vi "MHM Get DLL Version.vi"(8 "error in (no error)":errorcluster) -> (0 "error out":errorcluster, 2 "pulDllVersion":u32[](array[numeric]), 3 "function return":u32)   [LabVIEW 2019, in "MHM_1SL_interface.lvlib"]
uses:
  MHM_1SL_interface.lvlib
  lib/MHM_1SL_interface.dll
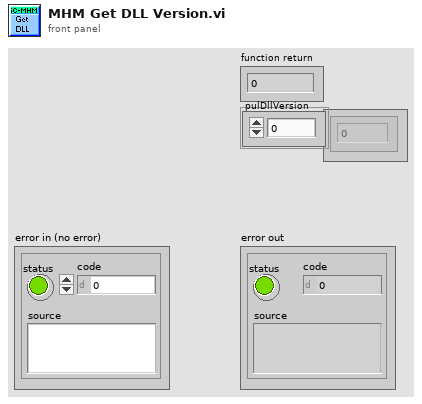
[diagram p1: front panel]
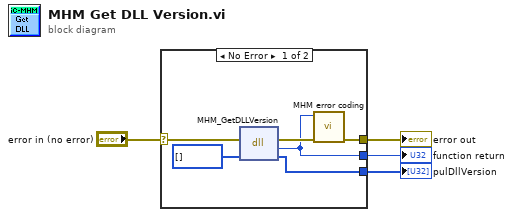
[diagram p0: block diagram]
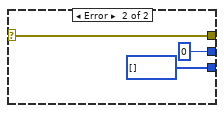
[diagram p2: hidden frame]
diagram:
  n1 = case shown="No Error" "error in (no error)" {
    selector: "error in (no error)" -> [w9 w13]
    tunnel: [w8 u32[] [] ("pulDllVersion")] -> w3
    tunnel: [w7 w13] -> w2
    tunnel: [w6 u32 0 ("return type")] -> w1
    frame No Error {
      n2 = dll-call lib="C:/workspace/project/scancon/MHM_1SL_interface_4.4.0/lv_interface/lib/MHM_1SL_interface.dll" fn="MHM_GetDLLVersion"(error in=w9, "pulDllVersion"=u32[] []) -> (error out=w10:errorcluster, "return type"=w6:u32, "pulDllVersion"=w8:u32[])  [unwired: 2 in, 1 out]
      n3 = call "MHM error coding.vi"("error in (no error)"=w10, "function return in"=w6) -> ("error out"=w7:errorcluster)  [unwired: 9 in]
    }
    frame Error {
    }
  }
  "error out" <- w2
  "function return" <- w1
  "pulDllVersion" <- w3
